vi "MainVI.vi"() -> ()   [LabVIEW 2022 SP3]
uses:
  <vilib>/MakerHub/LINX/Public/Sensors/Accelerometer/MPU60X0/DeviceAddresses.ctl
  <vilib>/MakerHub/LINX/Public/Sensors/Accelerometer/MPU60X0/Clock Source.ctl
  <vilib>/Analysis/3filter.llb/Filter Passband Type.ctl
  <vilib>/MakerHub/LINX/Public/Peripherals/Digital/Digital Write 1 Chan.vi
  <vilib>/DAQmx/read.llb/DAQmx Read (Analog 1D DBL NChan 1Samp).vi
  <vilib>/MakerHub/LINX/Public/Peripherals/Digital/Digital Write N Chans.vi
  <vilib>/MakerHub/LINX/Private/Local IO/LinxDigitalWrite.vi
  <vilib>/MakerHub/LINX/Public/Utilities/Check Channel.vi
  <vilib>/DAQmx/create/channels.llb/DAQmx Create Channel (AI-Voltage-Basic).vi
  <vilib>/smtpClient/Set Message Text.vi
  <vilib>/DAQmx/miscellaneous.llb/DAQmx Fill In Error Info.vi
  <vilib>/MakerHub/LINX/Public/Utilities/Open Serial.vi
  <vilib>/MakerHub/LINX/Private/Utilties/Generate Error.vi
  <vilib>/MakerHub/LINX/Public/Sensors/Accelerometer/MPU60X0/MPU60X0.lvlib
  <vilib>/MakerHub/LINX/LMH-LINX.lvlib
  <vilib>/smtpClient/LabVIEWSMTPClient.lvlib
  <vilib>/ptbypt/NI_PtbyPt.lvlib
  <vilib>/Analysis/NI_AALBase.lvlib
panel:
  out "Voltage":dbl
  out "Final Alert indicator":bool
  out "Force Output":dbl
  out "LED Alert":bool
  out "Force Sensor":string
  out "Alert from DAQ":bool
  in  "Serial Port":refnum<visa-resource-name>="N/A"
  out "Vibration Motor Alert":bool
  in  "Stop LINX":bool
  out "Alert Message":string
  out "Acceleration Data (g)":T1
  out "LM35 Sensor":string
  out "Temperature":dbl(graph)
  out "Thermometer":dbl(slide) scale=0.0..100.0
  out "Gas Sensor Waveform":dbl(knob) scale=0.0..3.0
  out "Gas Sensor":string
  in  "DAQmx Physical Channel":tag
  in  "Stop DAQ":bool
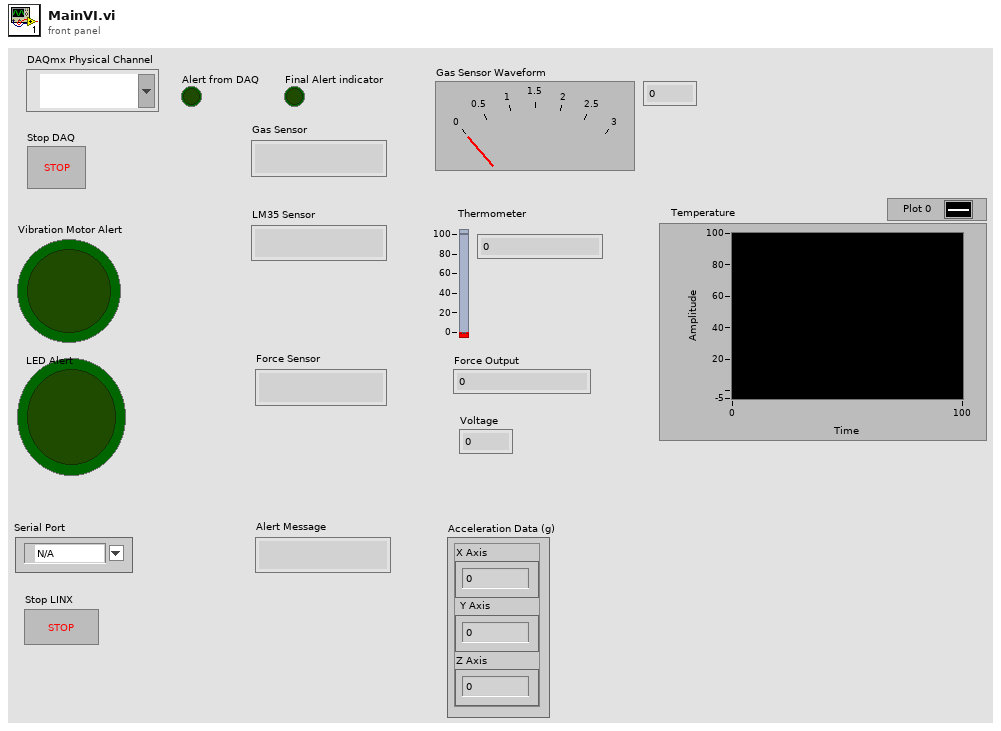
[diagram p1: front panel]
types:
  T1 = cluster{"X Axis":i16, "Y Axis":i16, "Z Axis":i16}
  T2 = typedef "LMH-LINX.lvlib/MPU60X0.lvlib/Clock Source.ctl" = enum8{"Internal 8MHz Osc", "PLL with X Gyro Ref", "PLL with Y Gyro Ref", "PLL with Z Gyro Ref", "PLL with ext 32.768 KHz Ref", "PLL with ext 19.2 MHz Ref", "Reserved", "Hold in reset"}
  T3 = typedef "LMH-LINX.lvlib/MPU60X0.lvlib/DeviceAddresses.ctl" = enum16{"0x68", "0x69"}
  T4 = typedef "LMH-LINX.lvlib/LINX Ref.ctl" = cluster{"IO":T5, "Interface":T6, "LINX Device Config":T7}
  T5 = typedef "LMH-LINX.lvlib/Platform.ctl" = enum16{"Remote", "Local"}
  T6 = typedef "LMH-LINX.lvlib/Interface.ctl" = enum16{"Serial", "TCP"}
  T7 = typedef "LMH-LINX.lvlib/Device.lvlib/LINX Device Config.ctl" = cluster{"Interface":T6, "COM Port":refnum<visa-resource-name>, "TCP Configuration":T8, "Device Family":u8, "Device ID":u8, "Device Name":string, "TCP Ref":refnum<k5>, "Channels":T9}
  T8 = typedef "LMH-LINX.lvlib/Device.lvlib/TCP Config.ctl" = cluster{"IP Address":string, "Port":u16}
  T9 = typedef "LMH-LINX.lvlib/Channels.ctl" = cluster{"DI":u8[], "DO":u8[], "AI":u8[], "AO":u8[], "PWM":u8[], "QE":u8[], "UART":u8[], "I2C 2":u8[], "SPI":u8[], "CAN":u8[], "Servo":u8[], "AI Ref (V)":dbl, "AI Resolution (Bits)":u8, "AO Ref (V)":dbl, "AO Resolution (Bits)":u8}
  T10 = typedef "NI_AALBase.lvlib/Filter Passband Type.ctl" = enum32{"Lowpass", "Highpass", "Bandpass", "Bandstop"}
  T11 = typedef "LabVIEWSMTPClient.lvlib/SmtpClientHandle.ctl" = refnum<k1>
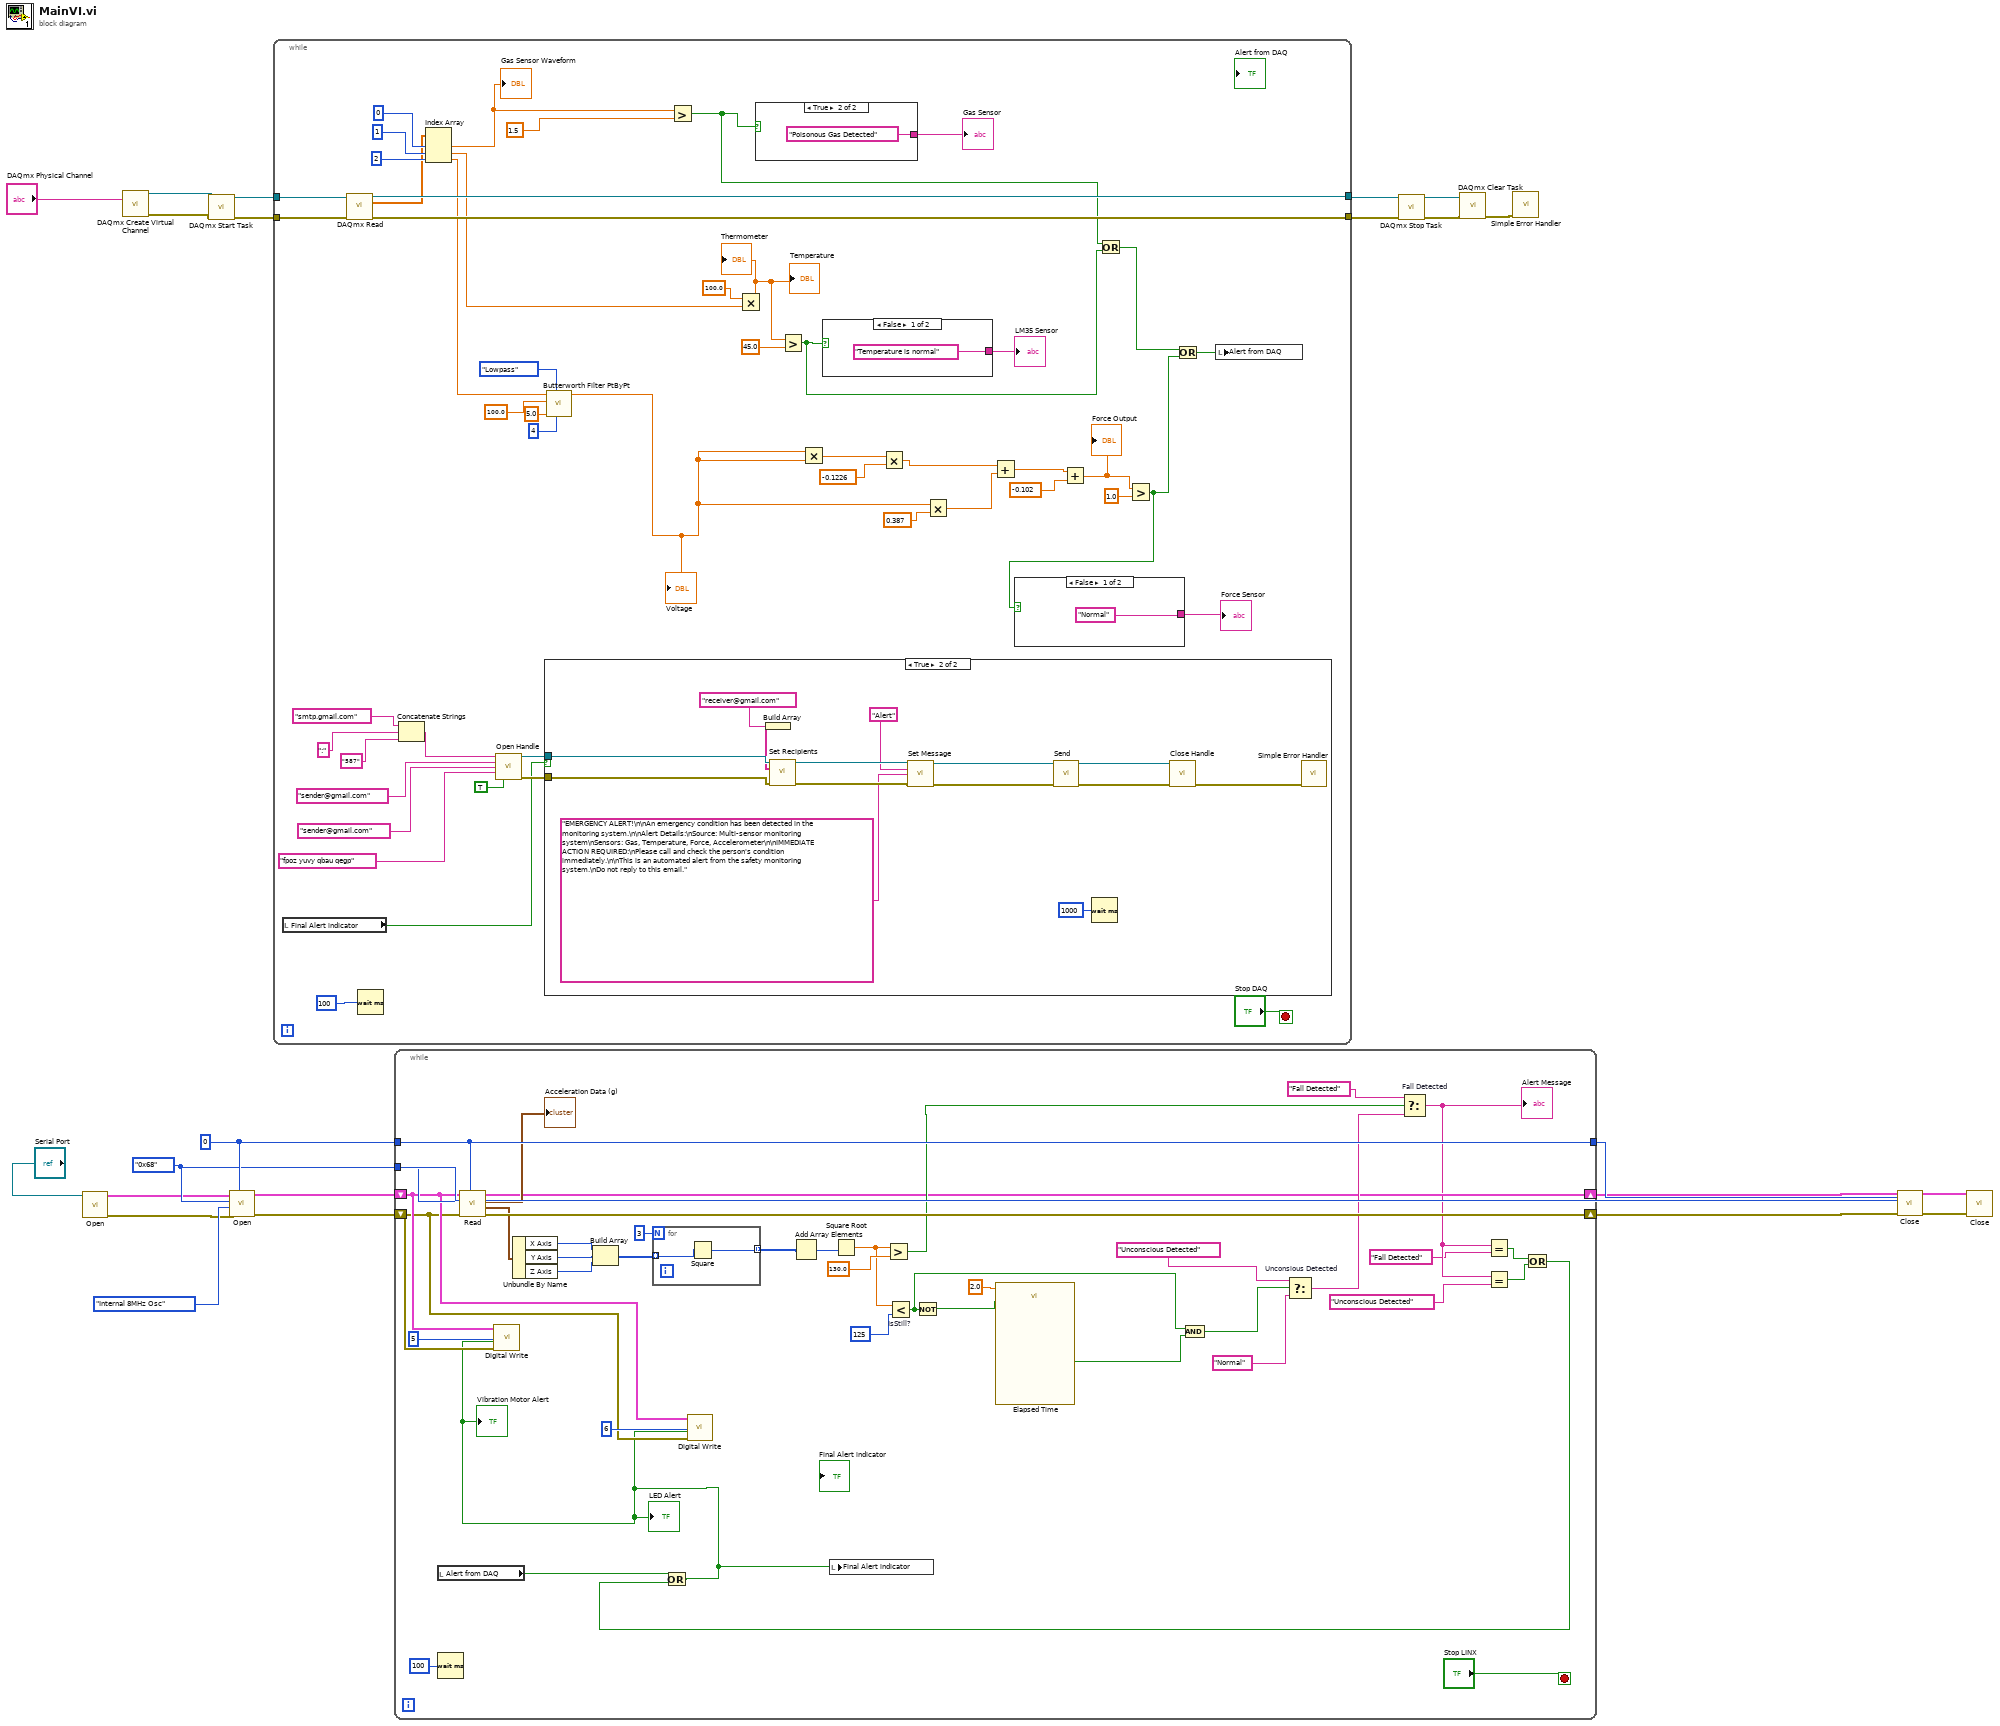
[diagram p0: block diagram]
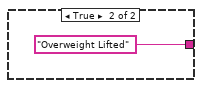
[diagram p3: hidden frame]
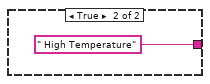
[diagram p4: hidden frame]
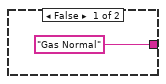
[diagram p5: hidden frame]
diagram:
  w9 = u8 0 ("I2C Channel")
  w8 = DeviceAddresses."0x68" ("I2C Slave Address")
  n1 = call-poly <vilib>:"Open.vi"("Serial Port"="Serial Port") -> ("Error Out"=w3:errorcluster, "LINX Resource"=w5:T4)  [unwired: 8 in, 1 out]
  n2 = call-poly <vilib>:"DAQmx Create Virtual Channel.vi"("physical channels"="DAQmx Physical Channel") -> ("task out"=w23:refnum<k21>, "error out"=w22:errorcluster)  [unwired: 13 in]
  n3 = call <vilib>:"DAQmx Start Task.vi"("task/channels in"=w23, "error in"=w22) -> ("task out"=w21:refnum<k21>, "error out"=w20:errorcluster)  [unwired: 12 in]
  n4 = call <vilib>:"Open.vi"("I2C Channel"=w9, "Error In"=w3, "Clock Source"=Clock_Source."Internal 8MHz Osc", "I2C Slave Address"=w8, "LINX Resource"=w5) -> ("Error Out"=w12:errorcluster, "LINX Resource"=w13:T4)  [unwired: 5 in]
  n5 = while {
    tunnel: w21 -> [w72]
    tunnel: w20 -> [w71]
    tunnel: [w70] -> w19
    tunnel: [w69] -> w18
    stop <- "Stop DAQ" stop-if-true
    n6 = local read "Final Alert indicator"() -> (w30:bool)
    n7 = call-poly <vilib>:"DAQmx Read.vi"("task/channels in"=w72, "error in"=w71) -> ("task out"=w70:refnum<k21>, "data"=w64:dbl[], "error out"=w69:errorcluster)  [unwired: 11 in]
    n8 = Wait (ms)(milliseconds to wait=u32 100) -> ()  [unwired: 1 out]
    n9 = Concatenate Strings("smtp.gmail.com", ":", "587") -> (w36:string)
    n10 = Index Array(array=w64, index #1=0 ("index"), index #2=1 ("index"), index #3=2 ("index")) -> (element #1=w61:dbl, element #2=w59:dbl, element #3=w25:dbl)
    "Gas Sensor Waveform" <- w61
    n11 = call <vilib>:"Open Handle.vi"("server address"=w36, "from"="sender@gmail.com", "username"="sender@gmail.com", "password"="fpoz yuvy qbau qegp", "use TLS (false)"=TRUE) -> ("handle out"=w41:T11, "error out"=w40:errorcluster)  [unwired: 9 in]
    n12 = case shown="True" w30 {
      tunnel: w41 -> [_ w87]
      tunnel: w40 -> [_ w83]
      frame False {
      }
      frame True {
        n13 = Build Array("receiver@gmail.com") -> (w78:string[])
        n14 = call <vilib>:"Set Recipients.vi"("handle in"=w87, "to"=w78, "error in (no error)"=w83) -> ("handle out"=w86:T11, "error out"=w82:errorcluster)  [unwired: 11 in]
        n15 = call-poly <vilib>:"Set Message.vi"("handle in"=w86, "subject"="Alert", "plain text message"="EMERGENCY ALERT!\n\nAn emergency condition has been detected in the monitoring system.\n\nAlert Details:\nSource: Multi-sensor monitoring system\nSensors: Gas, Temperature, Force, Accelerometer\n\nIMMEDIATE ACTION REQUIRED:\nPlease call and check the person's condition immediately.\n\nThis is an automated alert from the safety monitoring system.\nDo not reply to this email.", "error in (no error)"=w82) -> ("handle out"=w85:T11, "error out"=w81:errorcluster)  [unwired: 10 in]
        n16 = call <vilib>:"Send.vi"("handle in"=w85, "error in (no error)"=w81) -> ("handle out"=w84:T11, "error out"=w80:errorcluster)  [unwired: 11 in, 1 out]
        n17 = Wait (ms)(milliseconds to wait=u32 1000) -> ()  [unwired: 1 out]
        n18 = call <vilib>:"Close Handle.vi"("handle in"=w84, "error in (no error)"=w80) -> ("error out"=w75:errorcluster)  [unwired: 12 in, 1 out]
        n19 = call <vilib>:"Simple Error Handler.vi"("error in (no error)"=w75) -> ()  [unwired: 4 in, 5 out]
      }
    }
    n20 = call <vilib>:"Butterworth Filter PtByPt.vi"("order"=4, "filter type"=Filter_Passband_Type."Lowpass", "low cutoff freq: fl"=5.0, "sampling freq: fs"=100.0, "x"=w25) -> ("Filtered x"=w24:dbl)  [unwired: 4 in, 1 out]
    "Voltage" <- w24
    n21 = Greater?(x=w61, y=1.5) -> (0:w56:bool)
    n22 = Multiply(x=100.0, y=w59) -> (x*y=w58:dbl)
    "Thermometer" <- w58
    "Temperature" <- w58
    n23 = case shown="True" w56 {
      tunnel: ["Gas Normal" "Poisonous Gas Detected"] -> w62
      frame False {
      }
      frame True {
      }
    }
    "Gas Sensor" <- w62
    n24 = Greater?(x=w58, y=45.0) -> (0:w43:bool)
    n25 = Multiply(x=w24, y=w24) -> (x*y=w54:dbl)
    n26 = case shown="False" w43 {
      tunnel: ["Temperature is normal" " High Temperature"] -> w42
      frame False {
      }
      frame True {
      }
    }
    "LM35 Sensor" <- w42
    n27 = Multiply(x=w54, y=-0.1226) -> (x*y=w52:dbl)
    n28 = Multiply(x=w24, y=0.387) -> (x*y=w51:dbl)
    n29 = Add(x=w52, y=w51) -> (x+y=w50:dbl)
    n30 = Add(x=w50, y=-0.102) -> (x+y=w48:dbl)
    "Force Output" <- w48
    n31 = Or(x=w56, y=w43) -> (x .or. y?=w46:bool)
    n32 = Greater?(x=w48, y=1.0) -> (0:w45:bool)
    n33 = case shown="False" w45 {
      tunnel: ["Normal" "Overweight Lifted"] -> w44
      frame False {
      }
      frame True {
      }
    }
    "Force Sensor" <- w44
    n34 = Or(x=w46, y=w45) -> (x .or. y?=w32:bool)
    n35 = local write "Alert from DAQ"(w32) -> ()
  }
  n36 = while {
    tunnel: w9 -> [w129]
    tunnel: w8 -> [w132]
    shift-right: [w105] -> w2
    shift-left: w13 -> [w103]
    shift-right: [w133] -> w11
    shift-left: w12 -> [w102]
    tunnel: [w129] -> w6
    stop <- "Stop LINX" stop-if-true
    n37 = local read "Alert from DAQ"() -> (w95:bool)
    n38 = Wait (ms)(milliseconds to wait=u32 100) -> ()  [unwired: 1 out]
    n39 = call <vilib>:"Read.vi"("I2C Channel"=w129, "Error In"=w102, "I2C Slave Address"=w132, "LINX Resource"=w103) -> ("Error Out"=w133:errorcluster, "Gyro  Data (dps)"=w125:T1, "Acceleration Data (g)"=→"Acceleration Data (g)":T1, "LINX Resource"=w105:T4)  [unwired: 3 in, 1 out]
    n40 = Unbundle By Name(w125) -> ("X Axis"=w128:i16, "Y Axis"=w127:i16, "Z Axis"=w126:i16)
    n41 = Build Array(w128, w127, w126) -> (w121:i16[])
    n42 = for {
      N: 3 -> [_]
      tunnel: [w135] -> w123 mode=indexing
      tunnel: w121 -> [w134] mode=indexing
      n43 = Square(x=w134) -> (x^2=w135:i16)
    }
    n44 = Add Array Elements(numeric array=w123) -> (sum=w122:i16)
    n45 = Square Root(x=w122) -> (sqrt(x)=w118:dbl)
    n46 = Greater?(x=w118, y=130.0) -> (0:w111:bool)
    n47 = Less? "IsStill?"(x=w118, y=125) -> (x < y?=w106:bool)
    n48 = Not(x=w106) -> (.not. x?=w116:bool)
    n49 = call "Elapsed Time"("Time Target (s)"=2.0, "Reset"=w116) -> ("Time has Elapsed"=w115:bool)  [unwired: 10 in, 7 out]
    n50 = And(x=w106, y=w115) -> (x .and. y?=w114:bool)
    n51 = Select "Unconsious Detected"(t="Unconscious Detected", s=w114, f="Normal") -> (s? t:f=w109:string)
    n52 = Select "Fall Detected"(t="Fall Detected", s=w111, f=w109) -> (s? t:f=w101:string)
    "Alert Message" <- w101
    n53 = Equal?(x=w101, y="Fall Detected") -> (x = y?=w98:bool)
    n54 = Equal?(x=w101, y="Unconscious Detected") -> (x = y?=w97:bool)
    n55 = Or(x=w98, y=w97) -> (x .or. y?=w96:bool)
    n56 = Or(x=w95, y=w96) -> (x .or. y?=w94:bool)
    "Vibration Motor Alert" <- w94
    "LED Alert" <- w94
    n57 = call-poly <vilib>:"Digital Write.vi"("Error In"=w102, "Output Value"=w94, "DO Channel"=u8 5, "LINX Resource"=w103) -> ()  [unwired: 6 in, 2 out]
    n58 = call-poly <vilib>:"Digital Write.vi"("Error In"=w102, "Output Value"=w94, "DO Channel"=u8 6, "LINX Resource"=w103) -> ()  [unwired: 6 in, 2 out]
    n59 = local write "Final Alert indicator"(w94) -> ()
  }
  n60 = call <vilib>:"DAQmx Stop Task.vi"("task/channels in"=w19, "error in"=w18) -> ("task out"=w17:refnum<k21>, "error out"=w16:errorcluster)  [unwired: 12 in]
  n61 = call <vilib>:"DAQmx Clear Task.vi"("task in"=w17, "error in"=w16) -> ("error out"=w15:errorcluster)  [unwired: 13 in]
  n62 = call <vilib>:"Simple Error Handler.vi"("error in (no error)"=w15) -> ()  [unwired: 4 in, 5 out]
  n63 = call <vilib>:"Close.vi"("I2C Channel (0)"=w6, "Error In"=w11, "I2C Slave Address (0)"=w8, "LINX Resource"=w2) -> ("Error Out"=w7:errorcluster, "LINX Resource"=w4:T4)  [unwired: 6 in]
  n64 = call <vilib>:"Close.vi"("Error In"=w7, "LINX Resource"=w4) -> ()  [unwired: 9 in, 1 out]
